vi "Test Instrument Communications.vi"(8 "error in (no error)":errorcluster) -> (0 "error out":errorcluster)   [LabVIEW 2016, in "Hall Effect Library.lvlib"]
uses:
  Hall Effect Library.lvlib
  Private/Global Variables/Instrument Locations.vi
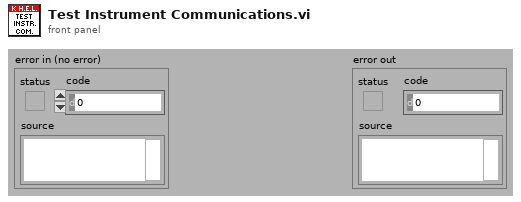
[diagram p1: front panel]
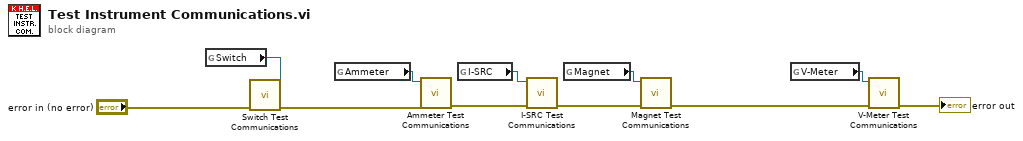
[diagram p0: block diagram]
diagram:
  n1 = global read "Instrument Locations.vi" "Switch"() -> (w5:refnum<visa-resource-name>)
  n2 = call "Switch Test Communications.vi"("error in (no error)"="error in (no error)", "VISA resource name in"=w5) -> ("error out"=w2:errorcluster)  [unwired: 9 out]
  n3 = global read "Instrument Locations.vi" "Ammeter"() -> (w8:refnum<visa-resource-name>)
  n4 = call "Ammeter Test Communications.vi"("error in (no error)"=w2, "VISA resource name in"=w8) -> ("error out"=w11:errorcluster)  [unwired: 9 out]
  n5 = global read "Instrument Locations.vi" "I-SRC"() -> (w7:refnum<visa-resource-name>)
  n6 = call "I-SRC Test Communications.vi"("error in (no error)"=w11, "VISA resource name in"=w7) -> ("error out"=w10:errorcluster)  [unwired: 9 out]
  n7 = global read "Instrument Locations.vi" "Magnet"() -> (w6:refnum<visa-resource-name>)
  n8 = call "Magnet Test Communications.vi"("error in (no error)"=w10, "VISA resource name in"=w6) -> ("error out"=w1:errorcluster)  [unwired: 9 out]
  n9 = global read "Instrument Locations.vi" "V-Meter"() -> (w4:refnum<visa-resource-name>)
  n10 = call "V-Meter Test Communications.vi"("error in (no error)"=w1, "VISA resource name in"=w4) -> ("error out"=→"error out":errorcluster)  [unwired: 9 out]
